vi "3_1_MNIST_Inference(CPU,GPU).vi"() -> ()   [LabVIEW 2020]
uses:
  <vilib>/Ngene/Deep Learning Toolkit/Toolkit/NN_Network/Controls/NN_Device.ctl
  <vilib>/Ngene/Deep Learning Toolkit/Toolkit/NN_Network/Controls/NN_Save_Before_Destroy_Options.ctl
  <extravilib>/ChannelInstances/Tag-bool/Write With Abort.vi
  <extravilib>/ChannelInstances/Tag-bool/Read With Abort.vi
  <extravilib>/ChannelInstances/Tag-bool/Instantiate.vi
  <extravilib>/ChannelInstances/Tag-bool/Endpoint.vi
  <extravilib>/ChannelInstances/Tag-bool/EndpointRead.vi
  <vilib>/Ngene/Deep Learning Toolkit/Toolkit/NN_Network/API/NN_Set_Input/3D/NN_Set_Input(3D_SGL_idx).vi
  <vilib>/Ngene/Deep Learning Toolkit/Toolkit/Deep_Learning_Toolkit_by_Ngene.lvlib
  <extravilib>/ChannelInstances/Tag-bool.lvlib
panel:
  in  "NN_Device":T1
  out "Labels":string[](array[string])=["0", "1", "2", "3", "4", "5", "6", "7", "8", "9"]
  in  "Network Configuration File Path":path=path "D:/Ngene/GitHub/deepltk_fpga_examples/1_MNIST_Classification(PXI,sbRIO)/Models/0_Original/MNIST_CNN/MNIST_CNN_net_cfg_24_11_25__15_33_35.cfg"
  in  "Weight File Path":path=path "D:/Ngene/GitHub/deepltk_fpga_examples/1_MNIST_Classification(PXI,sbRIO)/Models/0_Original/MNIST_CNN/MNIST_CNN_weights_24_11_25__15_33_35.bin"
  out "Pen Attributes":T2={"Width"=24, "Style"=enum."Solid"}
  out "Draw Digit (280x280 px)":picture
  in  "Pen Color":u32(colorbox)=197379
  in  "Stop":bool
  out "Test Speed (img/s)":dbl=390.7318407418141 format="%#_3p"
  out "test time(s/img)":dbl=0.0025592999999730637 format="%#_3p"
  out "Predictions":sgl[](array[slide])=[1.2135731e-08, 1.0, 2.7677905e-11, 4.1958145e-08, 2.4681273e-11, 2.9196653e-10, 2.7988944e-11, 4.588283e-08, 2.6504658e-11, 9.672841e-10] scale=0.0..1.0
  in  "Pen Width":dbl=24.0
  in  "Stop":bool
  out "image (28x28px)":sgl[][](graph)=[[-1.0, -1.0, -1.0, -1.0, -1.0, -1.0, -1.0, -1.0, -1.0, -1.0, -1.0, -1.0, -1.0, -1.0, -1.0, -1.0, -1.0, -1.0, -1.0, -1.0, -1.0, -1.0, -1.0, -1.0, -1.0, -1.0, -1.0, -1.0], [-1.0, -1.0, -1.0, -1.0, -1.0, -1.0, -1.0, -1.0, -1.0, -1.0, -1.0, -1.0, -1.0, -1.0, -1.0, -1.0, -1.0, -1.0, -1.0, -1.0, -1.0, -1.0, -1.0, -1.0, -1.0, -1.0, -1.0, -1.0], [-1.0, -1.0, -1.0, -1.0, -1.0, -1.0, -1.0, -1.0, -1.0, -1.0, -1.0, -1.0, -1.0, -1.0, -1.0, -1.0, -1.0, -1.0, -1.0, -1.0, -1.0, -1.0, -1.0, -1.0, -1.0, -1.0, -1.0, -1.0], [-1.0, -1.0, -1.0, -1.0, -1.0, -1.0, -1.0, -1.0, -1.0, -1.0, -1.0, -1.0, -1.0, -1.0, -1.0, -1.0, -1.0, -1.0, -1.0, -1.0, -1.0, -1.0, -1.0, -1.0, -1.0, -1.0, -1.0, -1.0], [-1.0, -1.0, -1.0, -1.0, -1.0, -1.0, -1.0, -1.0, -1.0, -1.0, -1.0, -1.0, -1.0, -1.0, -1.0, -1.0, -1.0, -1.0, -1.0, -1.0, -1.0, -1.0, -1.0, -1.0, -1.0, -1.0, -1.0, -1.0], [-1.0, -1.0, -1.0, -1.0, -1.0, -1.0, -1.0, -1.0, -1.0, -1.0, -1.0, -1.0, -1.0, -1.0, -1.0, -1.0, -1.0, -1.0, -1.0, -1.0, -1.0, -1.0, -1.0, -1.0, -1.0, -1.0, -1.0, -1.0], [-1.0, -1.0, -1.0, -1.0, -1.0, -1.0, -1.0, -1.0, -1.0, -1.0, -1.0, -1.0, -1.0, -1.0, -1.0, -1.0, -1.0, -1.0, -1.0, -1.0, -1.0, -1.0, -1.0, -1.0, -1.0, -1.0, -1.0, -1.0], [-1.0, -1.0, -1.0, -1.0, -1.0, -1.0, -1.0, -1.0, -1.0, -1.0, -1.0, -1.0, -1.0, -1.0, -1.0, -1.0, -1.0, -1.0, -1.0, -1.0, -1.0, -1.0, -1.0, -1.0, -1.0, -1.0, -1.0, -1.0], [-1.0, -1.0, -1.0, -1.0, -1.0, -1.0, -1.0, -1.0, -1.0, -1.0, -1.0, -1.0, -1.0, -1.0, -1.0, -1.0, -1.0, -1.0, -1.0, -1.0, -1.0, -1.0, -1.0, -1.0, -1.0, -1.0, -1.0, -1.0], [-1.0, -1.0, -1.0, -1.0, -1.0, -1.0, -1.0, -1.0, -1.0, -1.0, -1.0, -1.0, -1.0, -1.0, -1.0, -1.0, -1.0, -1.0, -1.0, -1.0, -1.0, -1.0, -1.0, -1.0, -1.0, -1.0, -1.0, -1.0], [-1.0, -1.0, -1.0, -1.0, -1.0, -1.0, -1.0, -1.0, -1.0, -1.0, -1.0, -1.0, -1.0, -1.0, -1.0, -1.0, -1.0, -1.0, -1.0, -1.0, -1.0, -1.0, -1.0, -1.0, -1.0, -1.0, -1.0, -1.0], [-1.0, -1.0, -1.0, -1.0, -1.0, -1.0, -1.0, -1.0, -1.0, -1.0, -1.0, -1.0, -1.0, -1.0, -1.0, -1.0, -1.0, -1.0, -1.0, -1.0, -1.0, -1.0, -1.0, -1.0, -1.0, -1.0, -1.0, -1.0], [-1.0, -1.0, -1.0, -1.0, -1.0, -1.0, -1.0, -1.0, -1.0, -1.0, -1.0, -1.0, -1.0, -1.0, -1.0, -1.0, -1.0, -1.0, -1.0, -1.0, -1.0, -1.0, -1.0, -1.0, -1.0, -1.0, -1.0, -1.0], [-1.0, -1.0, -1.0, -1.0, -1.0, -1.0, -1.0, -1.0, -1.0, -1.0, -1.0, -1.0, -1.0, -1.0, -1.0, -1.0, -1.0, -1.0, -1.0, -1.0, -1.0, -1.0, -1.0, -1.0, -1.0, -1.0, -1.0, -1.0], [-1.0, -1.0, -1.0, -1.0, -1.0, -1.0, -1.0, -1.0, -1.0, -1.0, -1.0, -1.0, -1.0, -1.0, -1.0, -1.0, -1.0, -1.0, -1.0, -1.0, -1.0, -1.0, -1.0, -1.0, -1.0, -1.0, -1.0, -1.0], [-1.0, -1.0, -1.0, -1.0, -1.0, -1.0, -1.0, -1.0, -1.0, -1.0, -1.0, -1.0, -1.0, -1.0, -1.0, -1.0, -1.0, -1.0, -1.0, -1.0, -1.0, -1.0, -1.0, -1.0, -1.0, -1.0, -1.0, -1.0], [-1.0, -1.0, -1.0, -1.0, -1.0, -1.0, -1.0, -1.0, -1.0, -1.0, -1.0, -1.0, -1.0, -1.0, -1.0, -1.0, -1.0, -1.0, -1.0, -1.0, -1.0, -1.0, -1.0, -1.0, -1.0, -1.0, -1.0, -1.0], [-1.0, -1.0, -1.0, -1.0, -1.0, -1.0, -1.0, -1.0, -1.0, -1.0, -1.0, -1.0, -1.0, -1.0, -1.0, -1.0, -1.0, -1.0, -1.0, -1.0, -1.0, -1.0, -1.0, -1.0, -1.0, -1.0, -1.0, -1.0], [-1.0, -1.0, -1.0, -1.0, -1.0, -1.0, -1.0, -1.0, -1.0, -1.0, -1.0, -1.0, -1.0, -1.0, -1.0, -1.0, -1.0, -1.0, -1.0, -1.0, -1.0, -1.0, -1.0, -1.0, -1.0, -1.0, -1.0, -1.0], [-1.0, -1.0, -1.0, -1.0, -1.0, -1.0, -1.0, -1.0, -1.0, -1.0, -1.0, -1.0, -1.0, -1.0, -1.0, -1.0, -1.0, -1.0, -1.0, -1.0, -1.0, -1.0, -1.0, -1.0, -1.0, -1.0, -1.0, -1.0], [-1.0, -1.0, -1.0, -1.0, -1.0, -1.0, -1.0, -1.0, -1.0, -1.0, -1.0, -1.0, -1.0, -1.0, -1.0, -1.0, -1.0, -1.0, -1.0, -1.0, -1.0, -1.0, -1.0, -1.0, -1.0, -1.0, -1.0, -1.0], [-1.0, -1.0, -1.0, -1.0, -1.0, -1.0, -1.0, -1.0, -1.0, -1.0, -1.0, -1.0, -1.0, -1.0, -1.0, -1.0, -1.0, -1.0, -1.0, -1.0, -1.0, -1.0, -1.0, -1.0, -1.0, -1.0, -1.0, -1.0], [-1.0, -1.0, -1.0, -1.0, -1.0, -1.0, -1.0, -1.0, -1.0, -1.0, -1.0, -1.0, -1.0, -1.0, -1.0, -1.0, -1.0, -1.0, -1.0, -1.0, -1.0, -1.0, -1.0, -1.0, -1.0, -1.0, -1.0, -1.0], [-1.0, -1.0, -1.0, -1.0, -1.0, -1.0, -1.0, -1.0, -1.0, -1.0, -1.0, -1.0, -1.0, -1.0, -1.0, -1.0, -1.0, -1.0, -1.0, -1.0, -1.0, -1.0, -1.0, -1.0, -1.0, -1.0, -1.0, -1.0], [-1.0, -1.0, -1.0, -1.0, -1.0, -1.0, -1.0, -1.0, -1.0, -1.0, -1.0, -1.0, -1.0, -1.0, -1.0, -1.0, -1.0, -1.0, -1.0, -1.0, -1.0, -1.0, -1.0, -1.0, -1.0, -1.0, -1.0, -1.0], [-1.0, -1.0, -1.0, -1.0, -1.0, -1.0, -1.0, -1.0, -1.0, -1.0, -1.0, -1.0, -1.0, -1.0, -1.0, -1.0, -1.0, -1.0, -1.0, -1.0, -1.0, -1.0, -1.0, -1.0, -1.0, -1.0, -1.0, -1.0], [-1.0, -1.0, -1.0, -1.0, -1.0, -1.0, -1.0, -1.0, -1.0, -1.0, -1.0, -1.0, -1.0, -1.0, -1.0, -1.0, -1.0, -1.0, -1.0, -1.0, -1.0, -1.0, -1.0, -1.0, -1.0, -1.0, -1.0, -1.0], [-1.0, -1.0, -1.0, -1.0, -1.0, -1.0, -1.0, -1.0, -1.0, -1.0, -1.0, -1.0, -1.0, -1.0, -1.0, -1.0, -1.0, -1.0, -1.0, -1.0, -1.0, -1.0, -1.0, -1.0, -1.0, -1.0, -1.0, -1.0]]
  # "Overview: This example demonstrates the usage of Deep Learning Toolkit for loading the model pre-trained for handwritten digit recognition and running for inference.\nRequirements: \nDeepLTK - Deep Learning Toolkit for LabVIEW (https://www.ngene.co/deep-learning-toolkit-for-labview)\nInstructions:\nThis example requires the training results (network topology file and trained weights file) generated by 0_MNIST(Train).vi\n1.\tProvide \"Network Configuration File Path\" and \"Weight File Path\" generated by 0_MNIST(Train).vi\n2.\tUse NN_Device to specify the device (CPU or GPU) for execution. GPU is applicable only for 64-bit LabVIEW.\n3.\tRun the VI.\n4.\tDraw a digit on the \"Draw Digit\" interface and observe the predictions results.\nMore Examples:  https://github.com/ngenehub/deepltk_examples"
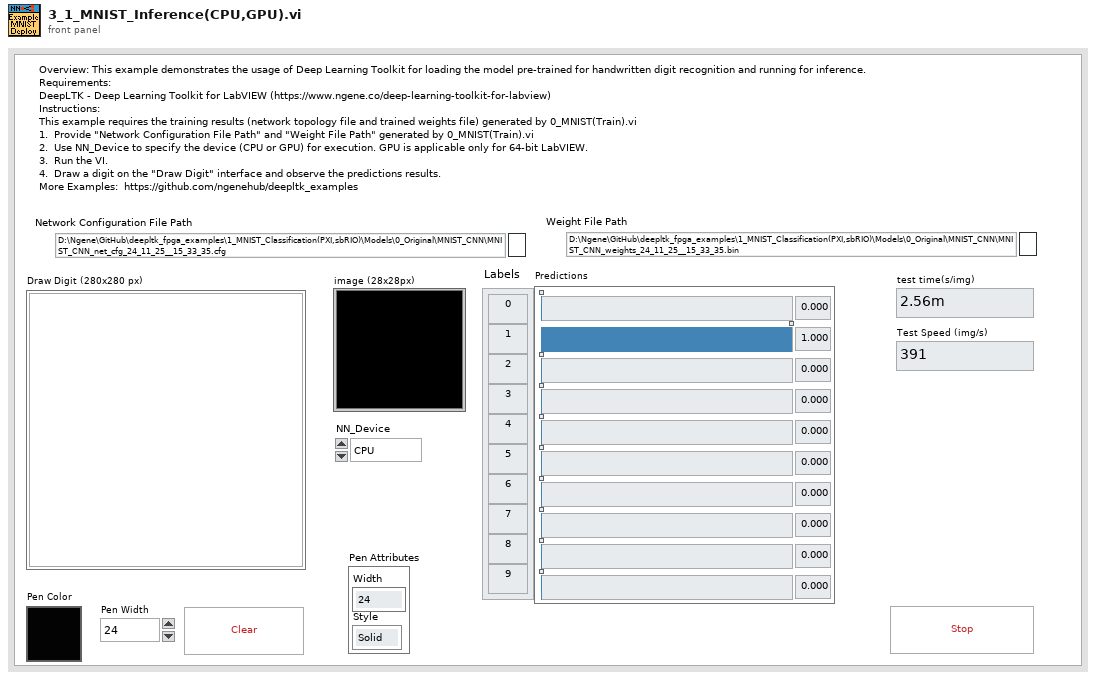
[diagram p1: front panel]
types:
  T1 = typedef "Deep_Learning_Toolkit_by_Ngene.lvlib/NN_Device.ctl" = enum16{"CPU", "GPU"}
  T2 = cluster{"Width":u16, "Style":enum32{"Solid", "Dash", "Dot", "DashDot", "DashDotDot"}}
  T3 = typedef "Deep_Learning_Toolkit_by_Ngene.lvlib/NN_Save_Before_Destroy_Options.ctl" = cluster{"CFG?":bool, "Weights?":bool, "Render?":bool}
  T4 = typedef "Deep_Learning_Toolkit_by_Ngene.lvlib/NN_Config_Params.ctl" = cluster{"Name":string, "mBatch":i32, "NN_Train_Params":T5, "LR_Decay_Policy":T8, "Labels":string[], "Loss":T10}
  T5 = typedef "Deep_Learning_Toolkit_by_Ngene.lvlib/NN_Train_Params.ctl" = cluster{"Optimizer":T6, "Beta_1":sgl, "Beta_2":sgl, "Weight Decay(L1)":sgl, "Weight Decay(L2)":sgl, "Data_Sampling":T7}
  T6 = typedef "Deep_Learning_Toolkit_by_Ngene.lvlib/NN_Train_Optimizer.ctl" = enum16{"SGD", "Adam", "Adagrad", "Adadelta", "RMSProp", "Nesterov"}
  T7 = typedef "Deep_Learning_Toolkit_by_Ngene.lvlib/NN_Train_Data_Sampling.ctl" = enum16{"Random", "Sequential"}
  T8 = typedef "Deep_Learning_Toolkit_by_Ngene.lvlib/NN_LR_Policy_Cfg.ctl" = cluster{"Policy_Type":T9, "LR0":dbl, "k":sgl, "WarmUp_Policy":enum16{"Step", "Ramp"}, "WarmUp_Iter":i32, "WarmUp_Ratio":sgl}
  T9 = typedef "Deep_Learning_Toolkit_by_Ngene.lvlib/NN_LR_Policy_Type.ctl" = enum16{"Manual", "Step", "Exp", "1/t"}
  T10 = typedef "Deep_Learning_Toolkit_by_Ngene.lvlib/NN_Loss_Config_Params.ctl" = cluster{"Loss_Type":T11, "Loss_Conf_Params":variant}
  T11 = typedef "Deep_Learning_Toolkit_by_Ngene.lvlib/NN_Loss_Type.ctl" = enum16{"None", "MSE", "CrossEntropy", "YOLO_v2", "YOLO_v4"}
  T12 = typedef "Deep_Learning_Toolkit_by_Ngene.lvlib/NN_Layer_Config_Params.ctl" = cluster{"Layer_Type":T13, "Layer_Conf_Params":variant, "Input Layers":string[]}
  T13 = typedef "Deep_Learning_Toolkit_by_Ngene.lvlib/NN_Layer_Type.ctl" = enum16{"Input1D", "Input3D", "Conv1D", "Conv2D", "Conv2D_Adv", "MaxPool", "AvgPool", "UpSample", "DropOut3D", "ShortCut", "Concat", "SoftMax3D", "FC", "DropOut", "Softmax", "Flatten", "YOLO_v2", "YOLO_v4", "Activation", "BatchNormalization", "Unsupported"}
  T14 = typedef "Deep_Learning_Toolkit_by_Ngene.lvlib/NN.ctl" = cluster{"Name":string, "No of Layers":i32, "mBatch":i32, "Layers":T15[], "Dimty":T16, "Dims_In":T17, "Dims_Out":T17, "Working_Dir":path, "Train?":bool, "Train_Params":T5, "LR_Update_Policy":T8, "Session Data":T18, "Ground_truth":T19, "NNg_hdls":T20, "NN_Device":T1, "GPU Id":i32, "Labels":string[], "Receptive Field":T21[], "Loss_Type":T11, "Loss_Cfg_Prms":variant, "NNG_WS":T22}
  T15 = typedef "Deep_Learning_Toolkit_by_Ngene.lvlib/NN_Layer_ref.ctl" = refnum<data-value>
  T16 = typedef "Deep_Learning_Toolkit_by_Ngene.lvlib/NN_In_Out_Dim-ty.ctl" = enum8{"In1D_Out1D", "In3D_Out1D", "In3D_Out3D", "In3D_OutBBox"}
  T17 = typedef "Deep_Learning_Toolkit_by_Ngene.lvlib/NN_Dims(C,H,W).ctl" = cluster{"C":i32, "H":i32, "W":i32}
  T18 = typedef "Deep_Learning_Toolkit_by_Ngene.lvlib/NN_Train_Session_Data.ctl" = cluster{"Epochs":sgl, "Tot_Iter":i32, "LR":sgl, "LR_iter":i32}
  T19 = typedef "Deep_Learning_Toolkit_by_Ngene.lvlib/NN_Ground_truth.ctl" = cluster{"Y":variant}
  T20 = typedef "Deep_Learning_Toolkit_by_Ngene.lvlib/nng_cuda_handles.ctl" = cluster{"cudnn":u64, "cublas":u64, "stream":u64, "curand":u64}
  T21 = typedef "Deep_Learning_Toolkit_by_Ngene.lvlib/NN_Dims(V,H).ctl" = cluster{"V":i32, "H":i32}
  T22 = typedef "Deep_Learning_Toolkit_by_Ngene.lvlib/NNG_WS.ctl" = cluster{"NNG_WS_Mem":T23, "Max_WS_Size":i64}
  T23 = typedef "Deep_Learning_Toolkit_by_Ngene.lvlib/NNg_WS_Mem_DVR.ctl" = refnum<data-value>
  T24 = cluster{"left":i16, "top":i16, "right":i16, "bottom":i16}
  T25 = typedef "LVMouseTypeDef.ctl" = cluster{"Mouse Position":cluster{"X":i32, "Y":i32}, "Mouse Modifiers":cluster{"Button Down":bool, "Shift Mod":bool, "Menu Mod":bool, "Option Mod":bool}}
  T26 = typedef "imagedata.ctl" = cluster{"image type":i32, "image depth":i32, "image":u8[], "mask":u8[], "colors":u32[], "Rectangle":cluster{"left":i16, "top":i16, "right":i16, "bottom":i16}}
  T27 = typedef "Tag-bool.lvlib/))Channel.ctl" = refnum<queue>
  T28 = typedef "Deep_Learning_Toolkit_by_Ngene.lvlib/NN_Layer.ctl" = cluster{"Name":string, "Layer_Data":variant, "Layer_Type":T13, "Dims_In":T17, "Layers_In":variant, "Dims_Out":T17, "Layers_Out":variant, "Metrics":T29, "GPU_Data":variant, "mBatch":i32, "NN_Device":T1, "NNg_hdls":T20, "Train?":bool, "Dimty":T30, "RecptField":T31}
  T29 = typedef "Deep_Learning_Toolkit_by_Ngene.lvlib/NN_Layer_Metrics.ctl" = cluster{"Data":dbl, "Params":dbl, "Ops":dbl}
  T30 = typedef "Deep_Learning_Toolkit_by_Ngene.lvlib/NN_Layer_Dimty.ctl" = enum16{"1D", "3D"}
  T31 = typedef "Deep_Learning_Toolkit_by_Ngene.lvlib/NN_Layer_RF_State.ctl" = cluster{"Dims":T21, "J":T21}
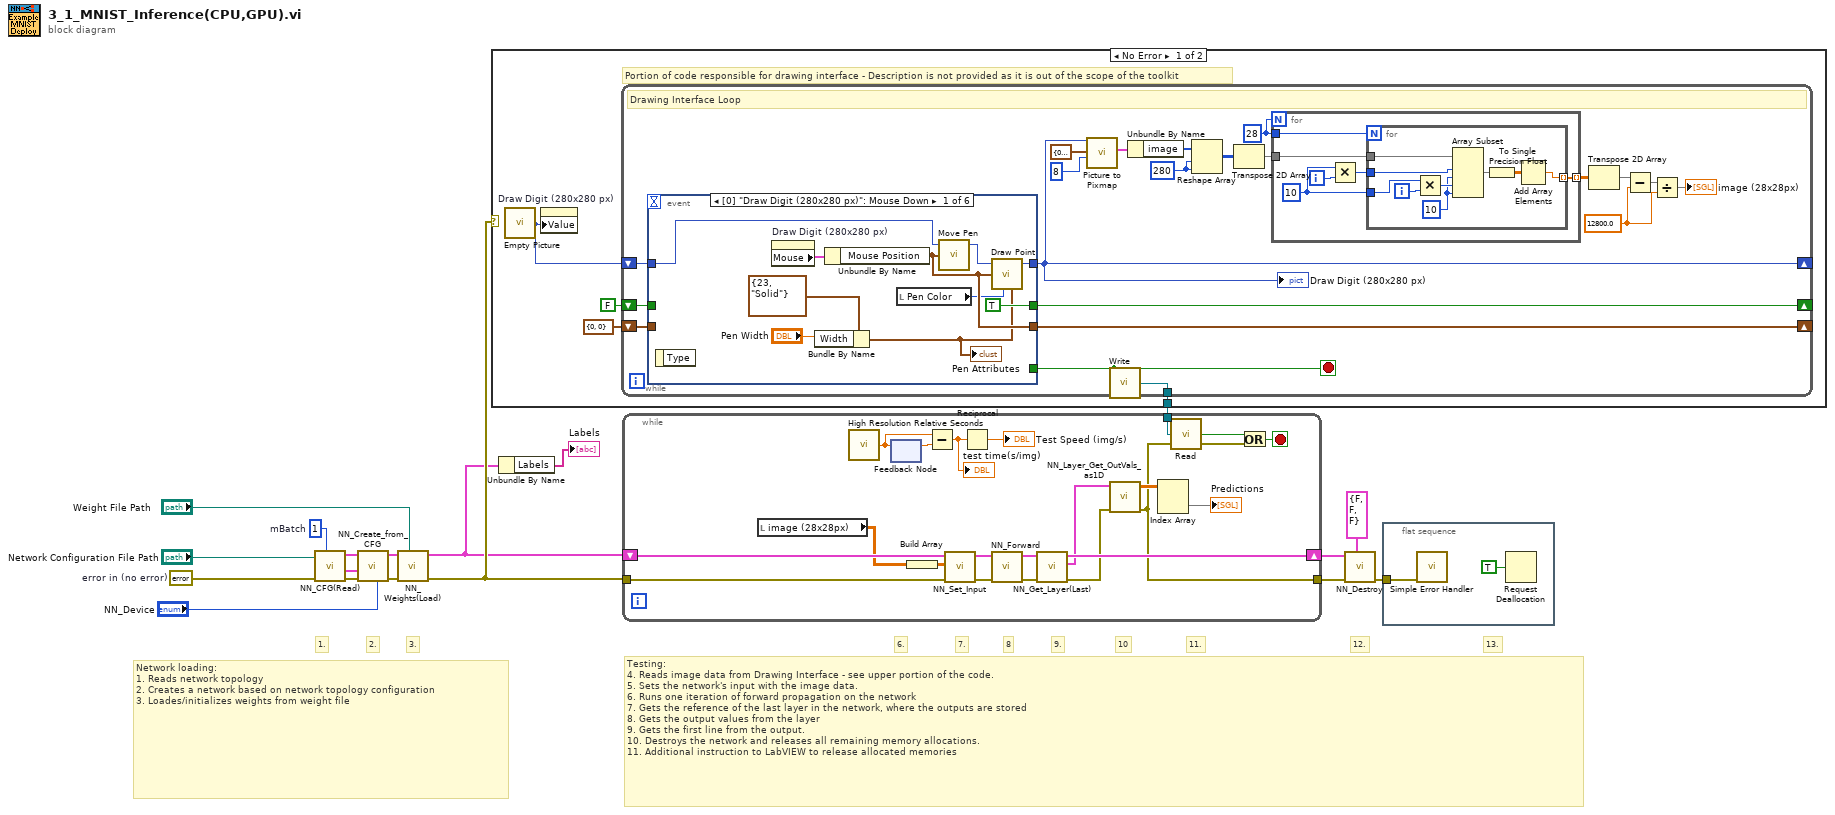
[diagram p0: block diagram]
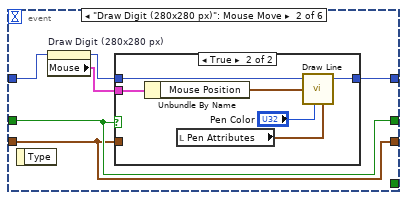
[diagram p2: hidden frame]
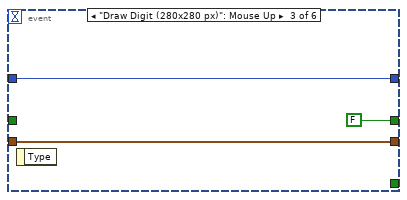
[diagram p4: hidden frame]
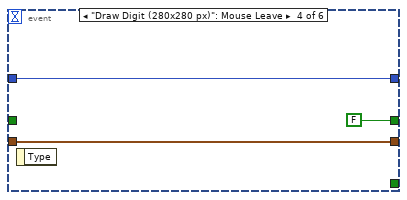
[diagram p5: hidden frame]
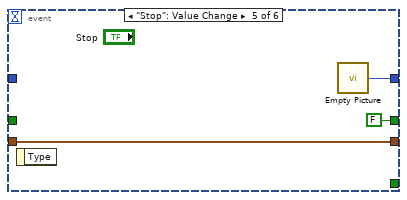
[diagram p6: hidden frame]
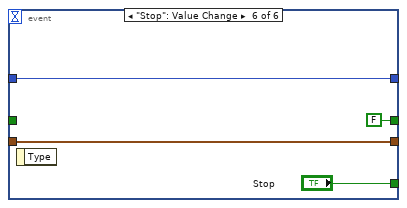
[diagram p7: hidden frame]
diagram:
  w6 = 1  # mBatch
  w13 = errorcluster {"status"=FALSE, "code"=0, "source"=""}  # error in (no error)
  # "Network loading:\n1.\tReads network topology\n2.\tCreates a network based on network topology configuration\n3.\tLoades/initializes weights from weight file"
  # "3."
  # "2."
  # "1."
  # "13."
  # "12."
  # "Testing:\n4.\tReads image data from Drawing Interface - see upper portion of the code.\n5.\tSets the network's input with the image data.\n6.\tRuns one iteration of forward propagation on the network\n7.\tGets the reference of the last layer in the network, where the outputs are stored\n8.\tGets the output values from the layer\n9.\tGets the first line from the output.\n10.\tDestroys the network and releases all remaining memory allocations.\n11.\tAdditional instruction to LabVIEW to release allocated memories"
  # "11."
  # "10"
  # "9."
  # "8"
  # "7."
  # "6."
  n1 = call <vilib>:"NN_CFG(Read).vi"("mBatch"=w6, "error in (no error)"=w13, "CFG file path"="Network Configuration File Path") -> ("error out"=w11:errorcluster, "Net_Cfg"=w12:T4, "Layer_Cfg"=w10:T12[])  [unwired: 6 in]
  n2 = call <vilib>:"NN_Create_from_CFG.vi"("NN_Device"="NN_Device", "error in (no error)"=w11, "Net_Cfg"=w12, "Layer_Cfg"=w10) -> ("error out"=w14:errorcluster, "NN out"=w9:T14)  [unwired: 6 in]
  n3 = call <vilib>:"NN_Weights(Load).vi"("Weight File Path"="Weight File Path", "error in (no error)"=w14, "NN in"=w9) -> ("error out"=w8:errorcluster, "NN out"=w5:T14)  [unwired: 7 in]
  n4 = case shown="No Error" w8 {
    tunnel: [w19 _] -> w7
    frame No Error {
      # "Portion of code responsible for drawing interface - Description is not provided as it is out of the scope of the toolkit"
      n5 = call "Empty Picture"() -> ("empty picture"=w22:picture)
      n6 = property on="Draw Digit (280x280 px)" class="Pict"("Value"=w22) -> ()  [unwired: 2 in, 2 out]
      n7 = while {
        shift-right: [w38] -> _
        shift-left: w22 -> [w43]
        shift-right: [w41] -> _
        shift-left: FALSE -> [w42]
        shift-right: [w39] -> _
        shift-left: cluster{"X":i32, "Y":i32} {"X"=0, "Y"=0} ("Mouse Position") -> [w40]
        tunnel: [w25] -> w19
        stop <- w30 stop-if-true
        w27 = sgl 12800.0 ("dimension size")
        w31 = 280 ("dimension size")
        w33 = 28
        # "Drawing Interface Loop"
        n8 = event shown="[0] \"Draw Digit (280x280 px)\": Mouse Down" {
          selector: _ -> [_ _ _ _ _ _]
          dyn-events: _ -> [_ _ _ _ _ _]
          timeout: _ -> [_ _ _ _ _ _]
          tunnel: [_ _ _ _ _ "Stop"] -> w30
          tunnel: [w65 w72 w83 w86 w89 w92] -> w38
          tunnel: w43 -> [w67 w71 w83 w86 _ w92]
          tunnel: w42 -> [_ w70 _ _ _ _]
          tunnel: [TRUE w70 FALSE FALSE FALSE FALSE] -> w41
          tunnel: w40 -> [_ w69 w81 w85 w88 w91]
          tunnel: [w63 w69 w81 w85 w88 w91] -> w39
          event "Draw Digit (280x280 px)": Mouse Down {
            # "Set the pen position, and draw an initial point or line."
            n9 = event-data() -> ()  [unwired: 1 in, 1 out]
            n10 = property on="Draw Digit (280x280 px)" class="Pict"() -> ("Mouse"=w68:T25)  [unwired: 2 in, 2 out]
            n11 = Bundle By Name(cluster=T2 {"Width"=23, "Style"=enum."Solid"} ("Pen Attributes"), "Width"="Pen Width") -> (w59:T2)
            "Pen Attributes" <- w59
            n12 = Unbundle By Name(w68) -> ("Mouse Position"=w63:cluster{"X":i32, "Y":i32})
            n13 = local read "Pen Color"() -> (w62:u32)
            n14 = call <vilib>:"Move Pen.vi"("new position"=w63, "picture"=w67) -> ("new picture"=w66:picture)  [unwired: 3 in]
            n15 = call <vilib>:"Draw Point.vi"("picture"=w66, "point(x,y)"=w63, "color(black)"=w62, "pen"=w59) -> ("new picture"=w65:picture)  [unwired: 5 in]
          }
          event "Draw Digit (280x280 px)": Mouse Move {
            # "Only draw if a Mouse Down event has occurred, but not a Mouse Up. Then, determine if the user is Drawing a point, a line, or selecting a subset and perform those operations in the case structure."
            n16 = event-data() -> ()  [unwired: 1 in, 1 out]
            n17 = property on="Draw Digit (280x280 px)" class="Pict"() -> ("Mouse"=w73:T25)  [unwired: 2 in, 2 out]
            n18 = case shown="True" w70 {
              tunnel: w71 -> [w74 w80]
              tunnel: w73 -> [_ w79]
              tunnel: [w74 w77] -> w72
              tunnel: w69 -> [_ _]
              frame False {
              }
              frame True {
                n19 = Unbundle By Name(w79) -> ("Mouse Position"=w78:cluster{"X":i32, "Y":i32})
                n20 = local read "Pen Attributes"() -> (w76:T2)
                n21 = call <vilib>:"Draw Line.vi"("picture"=w80, "end point"=w78, "color(black)"="Pen Color", "pen"=w76) -> ("new picture"=w77:picture)  [unwired: 5 in]
              }
            }
          }
          event "Draw Digit (280x280 px)": Mouse Up {
            # "When the user is finished drawing, we complete the operation. The only operation that we need to complete the Select Subset operation."
            n22 = event-data() -> ()  [unwired: 1 in, 1 out]
          }
          event "Draw Digit (280x280 px)": Mouse Leave {
            # "Change to the default cursor when the mouse leaves the picture."
            n23 = event-data() -> ()  [unwired: 1 in, 1 out]
          }
          event "Stop": Value Change {
            # "Erase the picture."
            n24 = event-data() -> ()  [unwired: 1 in, 1 out]
            n25 = call "Empty Picture"() -> ("empty picture"=w89:picture)
          }
          event "Stop": Value Change {
            # "Stop the VI."
            n26 = event-data() -> ()  [unwired: 1 in, 1 out]
          }
        }
        "Draw Digit (280x280 px)" <- w38
        n27 = call <vilib>:"Picture to Pixmap.vi"("depth"=8, "rect"=T24 {"left"=0, "top"=0, "right"=280, "bottom"=280}, "picture"=w38) -> ("image data"=w37:T26)  [unwired: 7 in, 1 out]
        n28 = call <extravilib>:"Write.vi"("element"=w30) -> ("channel"=w25:T27)  [unwired: 1 out]
        n29 = Unbundle By Name(w37) -> ("image"=w36:u8[])
        n30 = Reshape Array(w36, w31, w31) -> (w35:u8[][])
        n31 = Transpose 2D Array(2D array=w35) -> (transposed array=w34:u8[][])
        n32 = for {
          N: w33 -> [_]
          tunnel: w34 -> [w49]
          tunnel: w33 -> [w48]
          tunnel: [w44] -> w32 mode=indexing
          i -> [w47]
          w45 = 10 ("x")
          n33 = Multiply(x=w45, y=w47) -> (x*y=w46:i32)
          n34 = for {
            N: w48 -> [_]
            tunnel: w49 -> [w58]
            tunnel: w46 -> [w57]
            tunnel: w45 -> [w54]
            tunnel: [w50] -> w44 mode=indexing
            i -> [w56]
            w53 = 10 ("length")
            n35 = Multiply(x=w54, y=w56) -> (x*y=w55:i32)
            n36 = Array Subset(array=w58, index (row)=w57, length (row)=w53, index (col)=w55, length (col)=w53) -> (w52:u8[][])
            n37 = To Single Precision Float(number=w52) -> (single precision float=w51:sgl[][])
            n38 = Add Array Elements(numeric array=w51) -> (sum=w50:sgl)
          }
        }
        n39 = Transpose 2D Array(2D array=w32) -> (transposed array=w28:sgl[][])
        n40 = Subtract(x=w28, y=w27) -> (x-y=w29:sgl[][])
        n41 = Divide(x=w29, y=w27) -> (x/y=→"image (28x28px)":sgl[][])
      }
    }
    frame Error {
    }
  }
  n42 = Unbundle By Name(w5) -> ("Labels"=→"Labels":string[])
  n43 = while {
    shift-right: [w113] -> w17
    shift-left: w5 -> [w106]
    tunnel: w8 -> [w104]
    tunnel: [w97] -> w16
    tunnel: w7 -> [w96]
    stop <- w111 stop-if-true
    n44 = local read "image (28x28px)"() -> (w102:sgl[][])
    n45 = call <vilib>:"High Resolution Relative Seconds.vi"() -> ("relative seconds"=w109:dbl)
    n46 = feedback #1() -> (w110:dbl)  [unwired: 1 in]
    n47 = feedback-in #1(w109) -> ()
    n48 = Build Array(w102) -> (w94:sgl[][][])
    n49 = Subtract(x=w109, y=w110) -> (x-y=w108:dbl)
    "test time(s/img)" <- w108
    n50 = call-poly <vilib>:"NN_Set_Input.vi"("error in (no error)"=w104, "Data_In(3D_SGL)"=w94, "NN in"=w106) -> ("error out"=w103:errorcluster, "NN out"=w105:T14)  [unwired: 7 in]
    n51 = Reciprocal(x=w108) -> (1/x=→"Test Speed (img/s)":dbl)
    n52 = call <vilib>:"NN_Forward.vi"("error in (no error)"=w103, "NN in"=w105) -> ("error out"=w112:errorcluster, "NN out"=w114:T14)  [unwired: 6 in, 2 out]
    n53 = call <vilib>:"NN_Get_Layer(Last).vi"("error in (no error)"=w112, "NN in"=w114) -> ("error out"=w98:errorcluster, "Last_Layer"=w101:T28, "NN out"=w113:T14)  [unwired: 6 in, 1 out]
    n54 = call <vilib>:"NN_Layer_Get_OutVals_as1D.vi"("error in (no error)"=w98, "Layer"=w101) -> ("error out"=w97:errorcluster, "Out(as1D)"=w100:sgl[][])  [unwired: 8 in]
    n55 = Index Array(array=w100) -> (element=→"Predictions":sgl[])  [unwired: 2 in]
    n56 = call <extravilib>:"Read.vi"("channel"=w96) -> ("element"=w95:bool)  [unwired: 1 in, 1 out]
    n57 = Or(x=w95, y=w97) -> (x .or. y?=w111:bool)
  }
  n58 = call <vilib>:"NN_Destroy.vi"("Save (T, T, T)"=T3 {"CFG?"=FALSE, "Weights?"=FALSE, "Render?"=FALSE} ("Save_Config"), "error in (no error)"=w16, "NN in"=w17) -> ("error out"=w18:errorcluster)  [unwired: 7 in, 1 out]
  n59 = flat-sequence {
    tunnel: w18 -> [w116]
    frame #0 {
      n60 = call <vilib>:"Simple Error Handler.vi"("error in (no error)"=w116) -> ()  [unwired: 4 in, 5 out]
      n61 = Request Deallocation(TRUE ("flag")) -> ()
    }
  }
